vi "sliderGetPosition.vi"() -> (0 "position":i32)   [LabVIEW 2017]
uses:
  <vilib>/Instr/_visa.llb/VISA Flush IO Buffer Mask.ctl
  globalDevices.vi
panel:
  out "Bytes at Port":u32
  out "substring":string
  out "read buffer":string
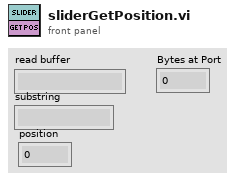
[diagram p1: front panel]
types:
  T1 = typedef "VISA Flush IO Buffer Mask.ctl" = u16
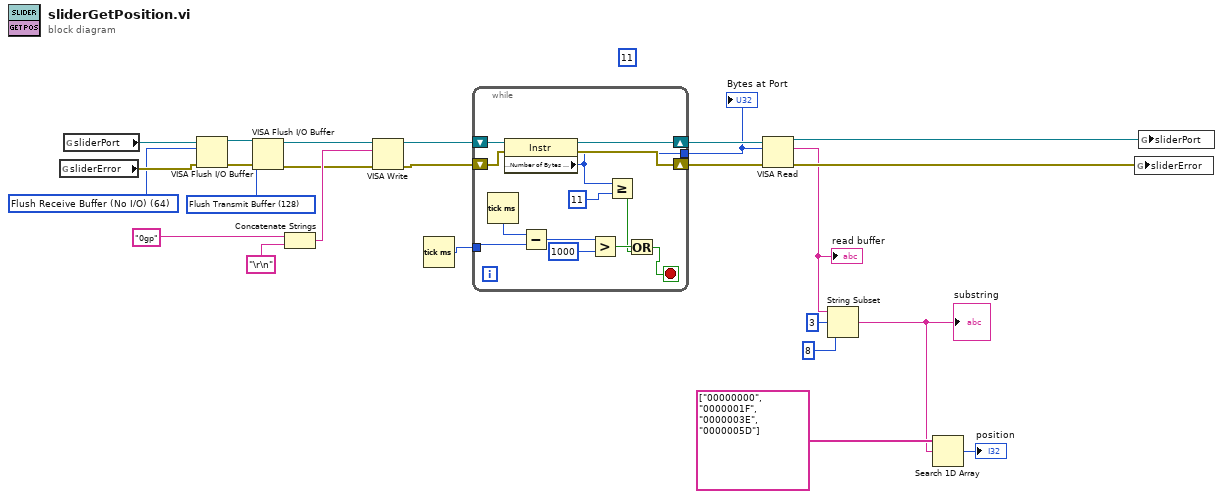
[diagram p0: block diagram]
diagram:
  w1 = T1 128 items=["Flush Receive Buffer"=16, "Write Transmit Buffer to Device"=32, "Flush Receive Buffer (No I/O)"=64, "Flush Transmit Buffer"=128] ("Mask")
  w6 = T1 64 items=["Flush Receive Buffer"=16, "Write Transmit Buffer to Device"=32, "Flush Receive Buffer (No I/O)"=64, "Flush Transmit Buffer"=128] ("Mask")
  (unwired) u32 11 ("byte count")
  n1 = global read "globalDevices.vi" "sliderError"() -> (w14:errorcluster)
  n2 = global read "globalDevices.vi" "sliderPort"() -> (w15:refnum<visa-resource-name>)
  n3 = VISA Flush I/O Buffer(VISA resource name=w15, mask (16)=w6, error in (no error)=w14) -> (VISA resource name out=w4:refnum<visa-resource-name>, error out=w5:errorcluster)
  n4 = VISA Flush I/O Buffer(VISA resource name=w4, mask (16)=w1, error in (no error)=w5) -> (VISA resource name out=w3:refnum<visa-resource-name>, error out=w2:errorcluster)
  n5 = Concatenate Strings("0gp", "\r\n" ("string")) -> (w22:string)
  n6 = VISA Write(VISA resource name=w3, write buffer=w22, error in (no error)=w2) -> (VISA resource name out=w13:refnum<visa-resource-name>, error out=w12:errorcluster)  [unwired: 1 out]
  n7 = Tick Count (ms)() -> (millisecond timer value=w7:u32)
  n8 = while {
    tunnel: [w34] -> w8
    shift-right: [w36] -> w11
    shift-left: w13 -> [w38]
    shift-right: [w35] -> w10
    shift-left: w12 -> [w37]
    tunnel: w7 -> [w31]
    stop <- w27 stop-if-true
    n9 = Tick Count (ms)() -> (millisecond timer value=w32:u32)
    n10 = property class="Instr"(reference=w38, error in=w37) -> (reference out=w36:refnum<visa-resource-name>, error out=w35:errorcluster, "Serial Settings:Number of Bytes at Serial Port"=w34:u32)
    n11 = Subtract(x=w32, y=w31) -> (x-y=w30:u32)
    n12 = Greater?(x=w30, y=u32 1000) -> (0:w28:bool)
    n13 = Greater Or Equal?(x=w34, y=u32 11) -> (x >= y?=w26:bool)
    n14 = Or(x=w28, y=w26) -> (x .or. y?=w27:bool)
  }
  "Bytes at Port" <- w8
  n15 = VISA Read(VISA resource name=w11, byte count=w8, error in (no error)=w10) -> (VISA resource name out=w25:refnum<visa-resource-name>, read buffer=w20:string, error out=w24:errorcluster)  [unwired: 1 out]
  "read buffer" <- w20
  n16 = String Subset(string=w20, offset (0)=3, length (rest)=8 ("length (rest)")) -> (substring=w17:string)
  "substring" <- w17
  n17 = Search 1D Array(1D array=string[] ["00000000", "0000001F", "0000003E", "0000005D"], element=w17) -> (index of element=→"position":i32)  [unwired: 1 in]
  n18 = global write "globalDevices.vi" "sliderError"(w24) -> ()
  n19 = global write "globalDevices.vi" "sliderPort"(w25) -> ()
